vi "BackupAndIntakeMoat.vi"   [LabVIEW 2015]
uses:
  ShiftGlobals.vi
  MotorPositionGlobals.vi
  RobotCode/TwoBallAutoGlobals.vi
types:
  T1 = typedef "WPI_MotorControlDeviceRef.ctl" = cluster{"DeviceStatus":errorcluster, "Type":T2, "PWM":cluster{"PWM Channel":T3, "DeadBand":T4}, "CAN":cluster{"Device Number":u8, "Control Mode":T5, "Semaphore":T6, "Max Vout":dbl, "TalonSRX Control Mode":T7}, "Invert":bool}
  T2 = typedef "WPI_MotorControlType.ctl" = enum16{"PWM", "CAN", "CANTalonSRX"}
  T3 = typedef "FPGA_DIOPWMChannel.ctl" = enum8{"PWM 0", "PWM 1", "PWM 2", "PWM 3", "PWM 4", "PWM 5", "PWM 6", "PWM 7", "PWM 8", "PWM 9", "PWM MXP 0", "PWM MXP 1", "PWM MXP 2", "PWM MXP 3", "PWM MXP 4", "PWM MXP 5", "PWM MXP 6", "PWM MXP 7", "PWM MXP 8", "PWM MXP 9", "Invalid"}
  T4 = typedef "WPI_PWMDeadband.ctl" = cluster{"Name":string, "maxPositivePwm":i32, "minPositivePwm":i32, "centerPwm":i32, "maxNegativePwm":i32, "minNegativePwm":i32, "angularRange":u16}
  T5 = typedef "WPI_CANJaguar_ControlMode.ctl" = enum8{"Percent VBus", "Current", "Speed", "Position", "Voltage"}
  T6 = typedef "Semaphore RefNum" = refnum<k1>
  T7 = typedef "WPI_CANTalonSRX_APIControlMode.ctl" = enum8{"Percent VBus", "Speed", "Position", "Slave", "Unchanged / Invalid", "Voltage Compensation", "Current", "Motion Profile"}
  T8 = typedef "WPI_CANTalonSRX_GlobalStatus.ctl" = cluster{"Applied Throttle":dbl, "Module Enabled":bool, "CAN Error":errorcluster, "Closed Loop Error":dbl, "Forward Limit Switch Closed":bool, "Reverse Limit Switch Closed":bool, "Sensor Position":dbl, "Sensor Velocity":dbl, "Current":dbl, "Sticky Fault - Over Temp":bool, "Sticky Fault - Under Voltage":bool, "Sticky Fault - Forward Limit":bool, "Sticky Fault - Reverse Limit":bool, "Sticky Fault - Forward Soft Limit":bool, "Sticky Fault - Reverse Soft Limit":bool, "Brake is Enabled":bool, "Encoder Position":dbl, "Encoder Velocity":dbl, "Encoder Index Count":dbl, "Encoder A Pin State":bool, "Encoder B Pin State":bool, "Encoder Index Pin State":bool, "Analog In":dbl, "Analog In Velocity":dbl, "Temperature (C)":dbl, "Battery Voltage":dbl, "Control 5 Is Supported":bool, "Current Profile Slot Select":dbl, "Pos Div 8":bool, "Vel Div 4":bool, "Pulse Width Position":i32, "Pulse Width Velocity":i32, "Pulse Width Rise To Rise (us)":i32, "Pulse Width Rise To Fall (us)":i32, "Mot Prof Active Is Under Run":bool, "Mot Prof Active Has Under Run":bool, "Mot Prof Active Is Last":bool, "Mot Prof Active Velocity Only":bool, "Mot Prof Active Is Valid":bool, "Mot Prof Buffer Is Full":bool, "Mot Prof Active Profile Slot Select":i32, "Mot Prof NextID":i32, "Mot Prof Count":i32, "Mot Prof Active Velocity":dbl, "Mot Prof Active Position":dbl, "Mot Prof Output Enable":i32}
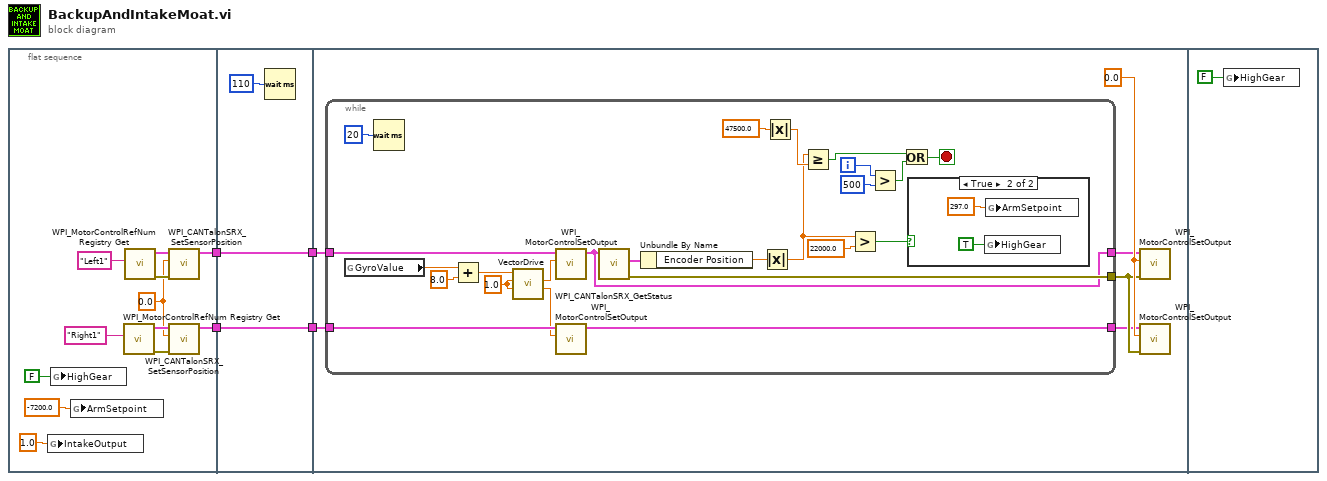
[diagram p0: block diagram]
diagram:
  n1 = flat-sequence {
    tunnel: [w9] -> w4
    tunnel: [w8] -> w3
    tunnel: w4 -> [w19]
    tunnel: [w19] -> w1
    tunnel: w3 -> [w18]
    tunnel: [w18] -> w2
    tunnel: w2 -> [w23]
    tunnel: w1 -> [w22]
    frame #0 {
      w10 = 0.0 ("New Sensor Position")
      n2 = global write "MotorPositionGlobals.vi" "IntakeOutput"(1.0 ("IntakeOutput")) -> ()
      n3 = global write "ShiftGlobals.vi" "HighGear"(FALSE ("HighGear")) -> ()
      n4 = global write "MotorPositionGlobals.vi" "ArmSetpoint"(-7200.0 ("ArmSetpoint")) -> ()
      n5 = call <vilib>:"WPI_MotorControlRefNum Registry Get.vi"("refnum name"="Right1") -> ("error out"=w14:errorcluster, "MotorControlDevRef"=w13:T1)  [unwired: 9 in]
      n6 = call <vilib>:"WPI_MotorControlRefNum Registry Get.vi"("refnum name"="Left1") -> ("error out"=w12:errorcluster, "MotorControlDevRef"=w11:T1)  [unwired: 9 in]
      n7 = call <vilib>:"WPI_CANTalonSRX_SetSensorPosition.vi"("error in (no error)"=w12, "New Sensor Position"=w10, "CAN Talon SRX Ref"=w11) -> ("CAN Talon SRX Ref"=w8:T1)  [unwired: 7 in, 1 out]
      n8 = call <vilib>:"WPI_CANTalonSRX_SetSensorPosition.vi"("error in (no error)"=w14, "New Sensor Position"=w10, "CAN Talon SRX Ref"=w13) -> ("CAN Talon SRX Ref"=w9:T1)  [unwired: 7 in, 1 out]
    }
    frame #1 {
      n9 = Wait (ms)(milliseconds to wait=u32 110) -> ()  [unwired: 1 out]
    }
    frame #2 {
      w25 = 0.0 ("Output")
      n10 = while {
        tunnel: [w39] -> w24
        tunnel: w23 -> [w38]
        tunnel: w22 -> [w37]
        tunnel: [w36] -> w21
        tunnel: [w35] -> w20
        i -> [w44]
        stop <- w46 stop-if-true
        w32 = 1.0 ("Output")
        n11 = global read "TwoBallAutoGlobals.vi" "GyroValue"() -> (w31:dbl)
        n12 = Wait (ms)(milliseconds to wait=u32 20) -> ()  [unwired: 1 out]
        n13 = Add(x=w31, y=8.0 ("setpoint")) -> (x+y=w29:dbl)
        n14 = call "VectorDrive.vi"("RightMotorInput"=w32, "LeftMotorInput"=w32, "setpoint"=w29) -> ("RightMotorOutput"=w33:dbl, "LeftMotorOutput"=w34:dbl)  [unwired: 7 in]
        n15 = call <vilib>:"WPI_MotorControlSetOutput.vi"("Output"=w34, "MotorControlDevRef"=w38) -> ("MotorControlDevRef"=w36:T1)  [unwired: 7 in, 2 out]
        n16 = call <vilib>:"WPI_MotorControlSetOutput.vi"("Output"=w33, "MotorControlDevRef"=w37) -> ("MotorControlDevRef"=w35:T1)  [unwired: 7 in, 2 out]
        n17 = call <vilib>:"WPI_CANTalonSRX_GetStatus.vi"("CAN Talon SRX Ref"=w36) -> ("error out"=w39:errorcluster, "Talon SRX Status"=w48:T8)  [unwired: 8 in, 1 out]
        n18 = Unbundle By Name(w48) -> ("Encoder Position"=w42:dbl)
        n19 = Absolute Value(x=w42) -> (abs(x)=w28:dbl)
        n20 = Absolute Value(x=47500.0) -> (abs(x)=w41:dbl)
        n21 = Greater Or Equal?(x=w28, y=w41) -> (x >= y?=w47:bool)
        n22 = Greater?(x=w28, y=22000.0) -> (0:w26:bool)
        n23 = Greater?(x=w44, y=500) -> (0:w45:bool)
        n24 = Or(x=w47, y=w45) -> (x .or. y?=w46:bool)
        n25 = case shown="True" w26 {
          frame False {
          }
          frame True {
            n26 = global write "ShiftGlobals.vi" "HighGear"(TRUE ("HighGear")) -> ()
            n27 = global write "MotorPositionGlobals.vi" "ArmSetpoint"(297.0 ("ArmSetpoint")) -> ()
          }
        }
      }
      n28 = call <vilib>:"WPI_MotorControlSetOutput.vi"("error in (no error)"=w24, "Output"=w25, "MotorControlDevRef"=w21) -> ()  [unwired: 6 in, 3 out]
      n29 = call <vilib>:"WPI_MotorControlSetOutput.vi"("error in (no error)"=w24, "Output"=w25, "MotorControlDevRef"=w20) -> ()  [unwired: 6 in, 3 out]
    }
    frame #3 {
      n30 = global write "ShiftGlobals.vi" "HighGear"(FALSE ("HighGear")) -> ()
    }
  }
